vi "Perform Step.vi"(8 "error in (no error)":errorcluster, 11 "Boolean Assertion in":refnum<class "Boolean Assertion.lvclass">) -> (0 "error out":errorcluster, 1 "Pass?":bool, 2 "Actual Value":variant, 3 "Boolean Assertion out":refnum<class "Boolean Assertion.lvclass">)   [LabVIEW 2020, in "MacroAssert.lvlib" / "Boolean Assertion.lvclass"]
doc: "Performs all actions required for <B>Step in</B>."
uses:
  Boolean Assertion.lvclass
  C:/Users/User/Documents/LabVIEW Data/Projects/MacroAssert/source/Classes/Assertion Step/Assertion Step.lvclass
  Boolean Assertion.lvclass/Boolean Assertion.ctl
  MacroAssert.lvlib
  SubVIs/Win Util/Win Util.lvlib
  SubVIs/Win Util/Window Refnum.ctl
  CTLs/FGV Actions.ctl
  SubVIs/Custom Errors/Custom Errors.lvlib
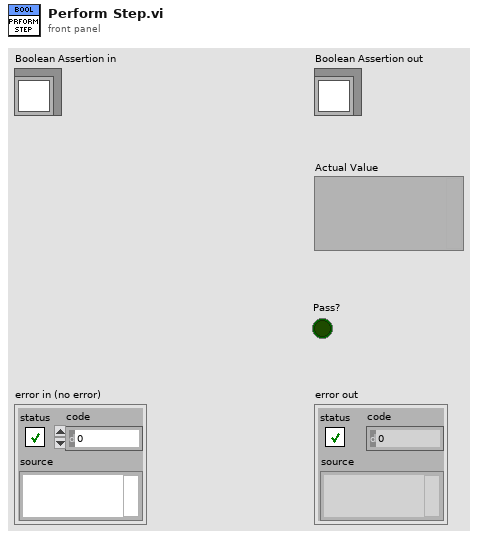
[diagram p1: front panel]
types:
  T1 = typedef "MacroAssert.lvlib/Boolean Assertion.lvclass/Boolean Assertion Type.ctl" = enum16{"Boolean Ctl Value", "Ctl Visible Property", "Ctl is Enabled", "Ctl is Grayed Out", "Ctl Key Focus Property", "VI Front Panel is Open", "Window is in Running Windows", "Window is in Monitor Bounds"}
  T2 = enum8{"Enabled", "Disabled", "Disabled and Grayed Out"}
  T3 = typedef "MacroAssert.lvlib/FGV Actions.ctl" = enum16{"Read", "Write"}
  T4 = typedef "MacroAssert.lvlib/Win Util.lvlib/Window Refnum.ctl" = u64
  T5 = enum32{"Invalid", "Standard", "Closed", "Hidden", "Minimized", "Maximized"}[]
  T6 = enum32{"Invalid", "Standard", "Closed", "Hidden", "Minimized", "Maximized"}
  T7 = cluster{"left":i16, "top":i16, "right":i16, "bottom":i16}
  T8 = cluster{"Left":i32, "Top":i32, "Right":i32, "Bottom":i32}[]
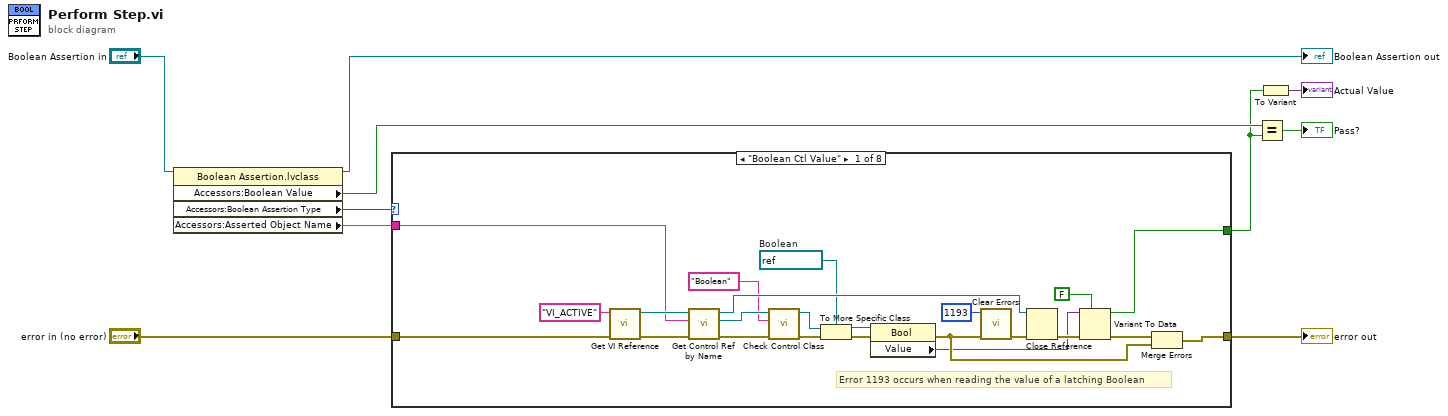
[diagram p0: block diagram]
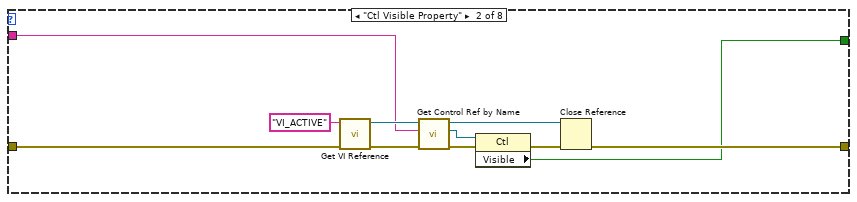
[diagram p2: hidden frame]
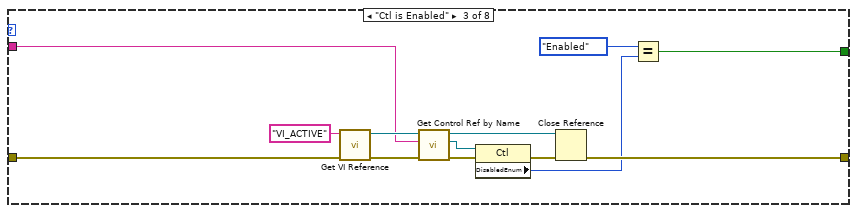
[diagram p3: hidden frame]
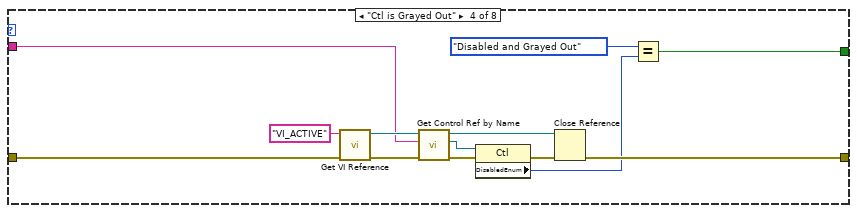
[diagram p4: hidden frame]
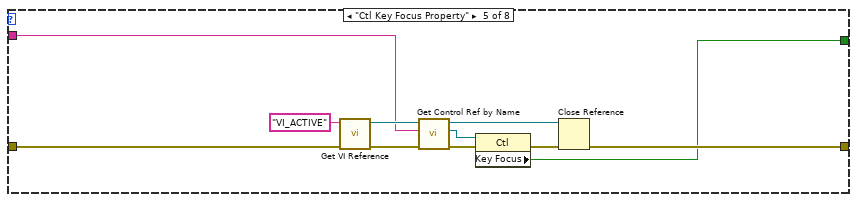
[diagram p5: hidden frame]
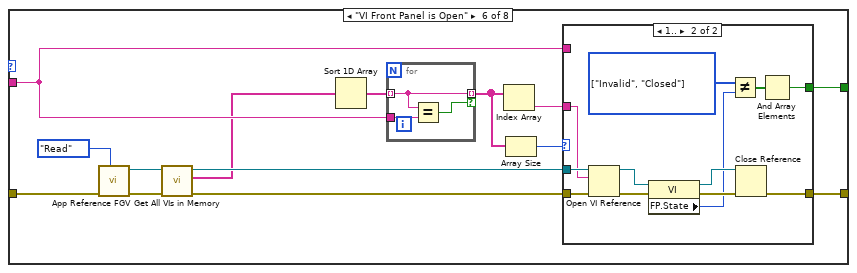
[diagram p6: hidden frame]
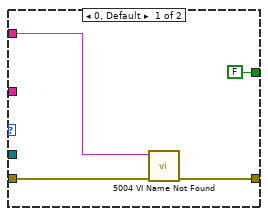
[diagram p7: hidden frame]
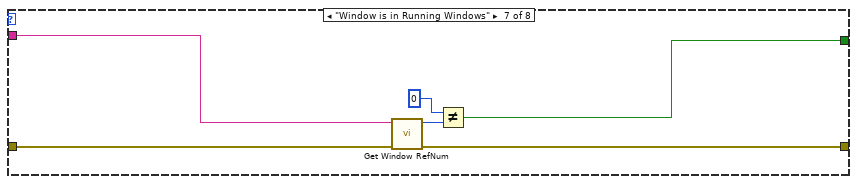
[diagram p8: hidden frame]
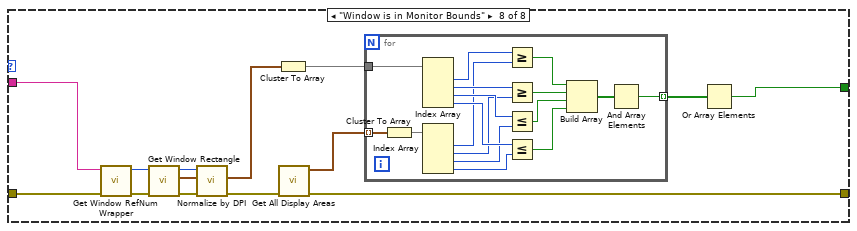
[diagram p9: hidden frame]
diagram:
  n1 = property class="Boolean Assertion.lvclass"(reference="Boolean Assertion in") -> (reference out=→"Boolean Assertion out":refnum<class "Boolean Assertion.lvclass">, "Accessors:Boolean Value"=w4:bool, "Accessors:Boolean Assertion Type"=w5:T1, "Accessors:Asserted Object Name"=w6:string)  [unwired: 1 in, 1 out]
  n2 = case shown="\"Boolean Ctl Value\"" w5 {
    tunnel: "error in (no error)" -> [w32 w42 w55 w68 w79 w94 w120 w134]
    tunnel: [w25 w40 w53 w66 w77 w95 w119 w131] -> w9
    tunnel: w6 -> [w17 w36 w49 w62 w73 w89 w118 w129]
    tunnel: [w14 w35 w46 w59 w72 w91 w115 w124] -> w3
    frame "Boolean Ctl Value" {
      w19 = refnum<vi> refnum  # Boolean
      # "Error 1193 occurs when reading the value of a latching Boolean"
      n3 = call "Get VI Reference.vi"("error in (no error)"=w32, "VI Name"="VI_ACTIVE") -> ("error out"=w33:errorcluster, "VI Ref"=w23:refnum<vi>)  [unwired: 8 in]
      n4 = call "Get Control Ref by Name.vi"("error in (no error)"=w33, "Name"=w17, "VI Ref"=w23) -> ("error out"=w30:errorcluster, "Ctl Ref"=w22:refnum<vi>, "VI Ref out"=w21:refnum<vi>)  [unwired: 6 in]
      n5 = call "Check Control Class.vi"("error in (no error)"=w30, "Supported Classes"="Boolean", "Ctl Ref"=w22) -> ("error out"=w29:errorcluster, "Ctl Ref out"=w20:refnum<vi>)  [unwired: 6 in, 1 out]
      n6 = To More Specific Class(target class=w19, reference=w20, error in=w29) -> (specific class reference=w18:refnum<vi>, error out=w27:errorcluster)
      n7 = property class="Bool"(reference=w18, error in=w27) -> (error out=w24:errorcluster, "Value"=w15:variant)  [unwired: 1 out]
      n8 = call <vilib>:"Clear Errors.vi"("error in (no error)"=w24, "specific error code to clear (0: all)"=1193) -> ("error out"=w26:errorcluster)  [unwired: 4 in, 1 out]
      n9 = Close Reference(reference=w21, error in (no error)=w26) -> (error out=w28:errorcluster)
      n10 = Variant To Data(error in=w28, type=FALSE, Variant=w15) -> (data=w14:bool, error out=w31:errorcluster)
      n11 = Merge Errors(w31, w24) -> (w25:errorcluster)
    }
    frame "Ctl Visible Property" {
      n12 = call "Get VI Reference.vi"("error in (no error)"=w42, "VI Name"="VI_ACTIVE") -> ("error out"=w44:errorcluster, "VI Ref"=w39:refnum<vi>)  [unwired: 8 in]
      n13 = call "Get Control Ref by Name.vi"("error in (no error)"=w44, "Name"=w36, "VI Ref"=w39) -> ("error out"=w43:errorcluster, "Ctl Ref"=w38:refnum<vi>, "VI Ref out"=w37:refnum<vi>)  [unwired: 6 in]
      n14 = property class="Ctl"(reference=w38, error in=w43) -> (error out=w41:errorcluster, "Visible"=w35:bool)  [unwired: 1 out]
      n15 = Close Reference(reference=w37, error in (no error)=w41) -> (error out=w40:errorcluster)
    }
    frame "Ctl is Enabled" {
      n16 = call "Get VI Reference.vi"("error in (no error)"=w55, "VI Name"="VI_ACTIVE") -> ("error out"=w57:errorcluster, "VI Ref"=w52:refnum<vi>)  [unwired: 8 in]
      n17 = call "Get Control Ref by Name.vi"("error in (no error)"=w57, "Name"=w49, "VI Ref"=w52) -> ("error out"=w56:errorcluster, "Ctl Ref"=w51:refnum<vi>, "VI Ref out"=w50:refnum<vi>)  [unwired: 6 in]
      n18 = property class="Ctl"(reference=w51, error in=w56) -> (error out=w54:errorcluster, "DisabledEnum"=w48:T2)  [unwired: 1 out]
      n19 = Close Reference(reference=w50, error in (no error)=w54) -> (error out=w53:errorcluster)
      n20 = Equal?(x=T2."Enabled", y=w48) -> (x = y?=w46:bool)
    }
    frame "Ctl is Grayed Out" {
      n21 = call "Get VI Reference.vi"("error in (no error)"=w68, "VI Name"="VI_ACTIVE") -> ("error out"=w70:errorcluster, "VI Ref"=w65:refnum<vi>)  [unwired: 8 in]
      n22 = call "Get Control Ref by Name.vi"("error in (no error)"=w70, "Name"=w62, "VI Ref"=w65) -> ("error out"=w69:errorcluster, "Ctl Ref"=w64:refnum<vi>, "VI Ref out"=w63:refnum<vi>)  [unwired: 6 in]
      n23 = property class="Ctl"(reference=w64, error in=w69) -> (error out=w67:errorcluster, "DisabledEnum"=w61:T2)  [unwired: 1 out]
      n24 = Close Reference(reference=w63, error in (no error)=w67) -> (error out=w66:errorcluster)
      n25 = Equal?(x=T2."Disabled and Grayed Out", y=w61) -> (x = y?=w59:bool)
    }
    frame "Ctl Key Focus Property" {
      n26 = call "Get VI Reference.vi"("error in (no error)"=w79, "VI Name"="VI_ACTIVE") -> ("error out"=w81:errorcluster, "VI Ref"=w76:refnum<vi>)  [unwired: 8 in]
      n27 = call "Get Control Ref by Name.vi"("error in (no error)"=w81, "Name"=w73, "VI Ref"=w76) -> ("error out"=w80:errorcluster, "Ctl Ref"=w75:refnum<vi>, "VI Ref out"=w74:refnum<vi>)  [unwired: 6 in]
      n28 = property class="Ctl"(reference=w75, error in=w80) -> (error out=w78:errorcluster, "Key Focus"=w72:bool)  [unwired: 1 out]
      n29 = Close Reference(reference=w74, error in (no error)=w78) -> (error out=w77:errorcluster)
    }
    frame "VI Front Panel is Open" {
      n30 = call "App Reference FGV.vi"("Mode"=FGV_Actions."Read", "error in (no error)"=w94) -> ("error out"=w86:errorcluster, "App Ref out"=w85:refnum<vi>)  [unwired: 8 in]
      n31 = call "Get All VIs in Memory.vi"("error in (no error)"=w86, "App Ref"=w85) -> ("error out"=w84:errorcluster, "All VIs in Memory"=w82:string[], "App Ref out"=w83:refnum<vi>)  [unwired: 7 in]
      n32 = Sort 1D Array(array=w82) -> (sorted array=w93:string[])
      n33 = for {
        tunnel: w93 -> [w113] mode=indexing
        tunnel: w89 -> [w114]
        tunnel: [w113] -> w92 mode=indexing if=w112
        n34 = Equal?(x=w113, y=w114) -> (x = y?=w112:bool)
      }
      n35 = Index Array(array=w92) -> (element=w88:string)  [unwired: 1 in]
      n36 = Array Size(array=w92) -> (size(s)=w87:i32)
      n37 = case shown="1.." w87 {
        tunnel: w88 -> [_ w104]
        tunnel: w84 -> [w98 w111]
        tunnel: [w97 w108] -> w95
        tunnel: [FALSE w100] -> w91
        tunnel: w83 -> [_ w106]
        tunnel: w89 -> [w96 _]
        frame 0, Default {
          n38 = call "5004 VI Name Not Found.vi"("error in (no error)"=w98, "VI Name"=w96) -> ("error out"=w97:errorcluster)  [unwired: 9 in]
        }
        frame 1.. {
          w102 = T5 [enum."Invalid", enum."Closed"] items=["Invalid", "Standard", "Closed", "Hidden", "Minimized", "Maximized"]
          n39 = Open VI Reference(application reference (local)=w106, vi path=w104, error in (no error)=w111) -> (vi reference=w107:refnum<vi>, error out=w110:errorcluster)  [unwired: 3 in]
          n40 = property class="VI"(reference=w107, error in=w110) -> (reference out=w105:refnum<vi>, error out=w109:errorcluster, "FP.State"=w103:T6)
          n41 = Not Equal?(x=w102, y=w103) -> (x != y?=w101:bool[])
          n42 = Close Reference(reference=w105, error in (no error)=w109) -> (error out=w108:errorcluster)
          n43 = And Array Elements(Boolean array=w101) -> (logical AND=w100:bool)
        }
      }
    }
    frame "Window is in Running Windows" {
      n44 = call "Get Window RefNum.vi"("error in (no error)"=w120, "window name (\"\")"=w118) -> ("error out"=w119:errorcluster, "window refnum (NaWR)"=w117:T4)  [unwired: 6 in]
      n45 = Not Equal?(x=T4 0 ("window refnum (NaWR)"), y=w117) -> (x != y?=w115:bool)
    }
    frame "Window is in Monitor Bounds" {
      n46 = call "Get Window RefNum Wrapper.vi"("error in (no error)"=w134, "Window Name"=w129) -> ("error out"=w132:errorcluster, "window refnum"=w127:T4)  [unwired: 8 in]
      n47 = call "Get Window Rectangle.vi"("error in (no error)"=w132, "window refnum (NaWR)"=w127) -> ("error out"=w133:errorcluster, "window rect"=w122:T7, "window refnum out"=w123:T4)  [unwired: 7 in]
      n48 = call "Normalize by DPI.vi"("error in (no error)"=w133, "window rect"=w122, "window refnum (NaWR)"=w123) -> ("error out"=w130:errorcluster, "normalized window rect"=w121:T7)  [unwired: 6 in, 1 out]
      n49 = Cluster To Array(cluster=w121) -> (array=w126:i16[])
      n50 = call "Get All Display Areas.vi"("error in (no error)"=w130) -> ("error out"=w131:errorcluster, "Display Areas"=w128:T8)  [unwired: 9 in]
      n51 = for {
        tunnel: w128 -> [w151] mode=indexing
        tunnel: w126 -> [w149]
        tunnel: [w135] -> w125 mode=indexing
        n52 = Cluster To Array(cluster=w151) -> (array=w150:i32[])
        n53 = Index Array(array=w149) -> (element #1=w148:i16, element #2=w147:i16, element #3=w146:i16, element #4=w145:i16)  [unwired: 4 in]
        n54 = Index Array(array=w150) -> (element #1=w144:i32, element #2=w143:i32, element #3=w142:i32, element #4=w141:i32)  [unwired: 4 in]
        n55 = Greater Or Equal?(x=w148, y=w144) -> (x >= y?=w140:bool)
        n56 = Greater Or Equal?(x=w147, y=w143) -> (x >= y?=w139:bool)
        n57 = Less Or Equal?(x=w146, y=w142) -> (x <= y?=w138:bool)
        n58 = Less Or Equal?(x=w145, y=w141) -> (x <= y?=w137:bool)
        n59 = Build Array(w140, w139, w138, w137) -> (w136:bool[])
        n60 = And Array Elements(Boolean array=w136) -> (logical AND=w135:bool)
      }
      n61 = Or Array Elements(Boolean array=w125) -> (logical OR=w124:bool)
    }
  }
  "error out" <- w9
  n62 = Equal?(x=w4, y=w3) -> (x = y?=→"Pass?":bool)
  n63 = To Variant(anything=w3) -> (Variant=→"Actual Value":variant)
